vi "控件启用与禁用.vi"(6 "启用效果(可选中)":enum16{"可选中", "不可选中"}(ring), 7 "禁用效果(变灰)":enum16{"变灰", "不可见"}(ring), 9 "启用？":bool, 11 "控件引用":refnum<vi>) -> (3 "引用输出":refnum<vi>)   [LabVIEW 2017]
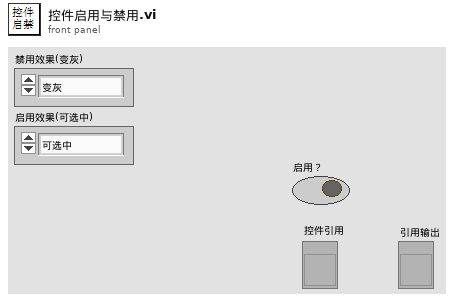
[diagram p1: front panel]
types:
  T1 = enum8{"Enabled", "Disabled", "Disabled and Grayed Out"}
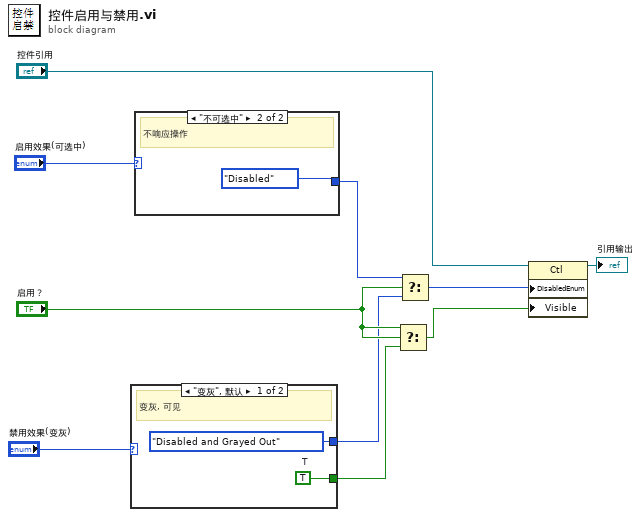
[diagram p0: block diagram]
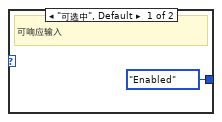
[diagram p2: hidden frame]
diagram:
  n1 = case shown="\"变灰\", 默认" "禁用效果(变灰)" {
    tunnel: [T1."Disabled and Grayed Out" ("禁用") _] -> w5
    tunnel: [w11 _] -> w4
    frame "变灰", Default {
      w11 = TRUE  # T
      # "变灰, 可见"
    }
    frame "不可见" {
      # "不可见"
    }
  }
  n2 = case shown="\"不可选中\"" "启用效果(可选中)" {
    tunnel: [T1."Enabled" ("禁用") T1."Disabled" ("禁用")] -> w1
    frame "可选中", Default {
      # "可响应输入"
    }
    frame "不可选中" {
      # "不响应操作"
    }
  }
  n3 = Select(t="启用？", s="启用？", f=w4) -> (s? t:f=w3:bool)
  n4 = Select(t=w1, s="启用？", f=w5) -> (s? t:f=w7:T1)
  n5 = property class="Ctl"(reference="控件引用", "DisabledEnum"=w7, "Visible"=w3) -> (reference out=→"引用输出":refnum<vi>)  [unwired: 1 in, 1 out]
